vi "MEMR-Get Preprocessed Data Filename.vi"(0 "Files":path[](array[path]), 5 "Threshold":T1) -> (8 "filename":path)   [LabVIEW 2020]
uses:
  MEMR-Offline Analysis Parameters.ctl
  <vilib>/regexp/Match Regular Expression.xnode
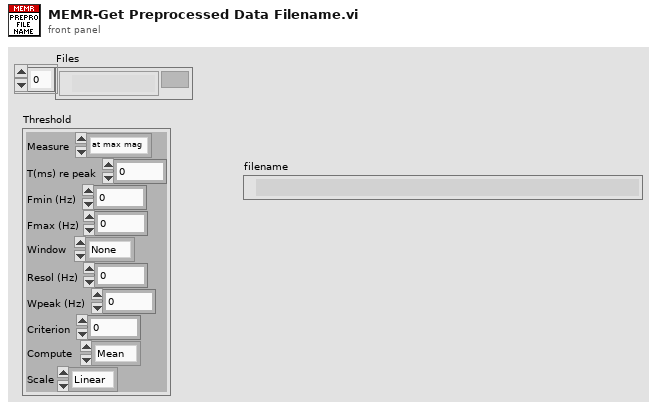
[diagram p1: front panel]
types:
  T1 = typedef "MEMR-Offline Analysis Parameters.ctl" = cluster{"Measure":enum16{"at max mag", "at max gain", "over window", "optimize", "Keefe"}, "T(ms) re peak":dbl, "Fmin (Hz)":dbl, "Fmax (Hz)":dbl, "Window":enum16{"None", "Hanning", "Hamming"}, "Resol (Hz)":dbl, "Wpeak (Hz)":dbl, "Criterion":dbl, "Compute":enum16{"Mean", "Sum"}, "Scale":enum16{"Linear", "Log"}}
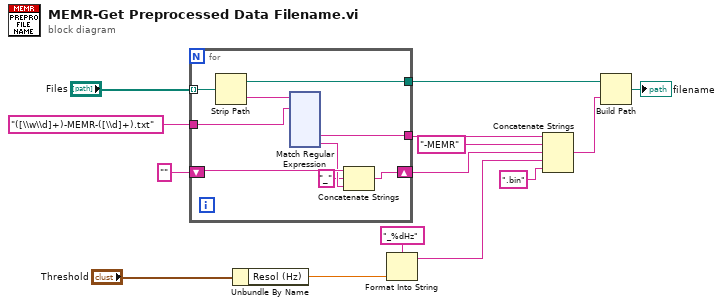
[diagram p0: block diagram]
diagram:
  n1 = for {
    tunnel: "Files" -> [w23] mode=indexing
    tunnel: "([\\w\\d]+)-MEMR-([\\d]+).txt" ("regular expression") -> [w21]
    tunnel: [w20] -> w11
    shift-right: [w19] -> w9
    shift-left: "" -> [w18]
    tunnel: [w15] -> w4
    n2 = Strip Path(path=w23) -> (stripped path=w15:path, name=w22:string)
    n3 = xnode "Match Regular Expression"("input string"=w22, "regular expression"=w21) -> ("submatch 1"=w20:string, "submatch 2"=w17:string)  [unwired: 4 in, 5 out]
    n4 = Concatenate Strings(w18, "_" ("string"), w17) -> (w19:string)
  }
  n5 = Unbundle By Name("Threshold") -> ("Resol (Hz)"=w7:dbl)
  n6 = Format Into String(format string="_%dHz", w7) -> (resulting string=w6:string)  [unwired: 2 in, 1 out]
  n7 = Concatenate Strings(w11, "-MEMR" ("string"), w9, w6, ".bin" ("string")) -> (w3:string)
  n8 = Build Path(base path=w4, name or relative path=w3) -> (appended path=→"filename":path)
